vi "sensor_parser.vi"(0 "Sensor configuration":string, 2 "error in":errorcluster) -> (3 "include_annotation":bool, 4 "Port out":u16, 5 "Stream dimensions":cluster{"x dimension":i32, "y dimension":i32}, 6 "error out":errorcluster)   [LabVIEW 2025]
doc: "Gets Sensor type and ports from the configuration text."
panel:
  out "Sensor":string
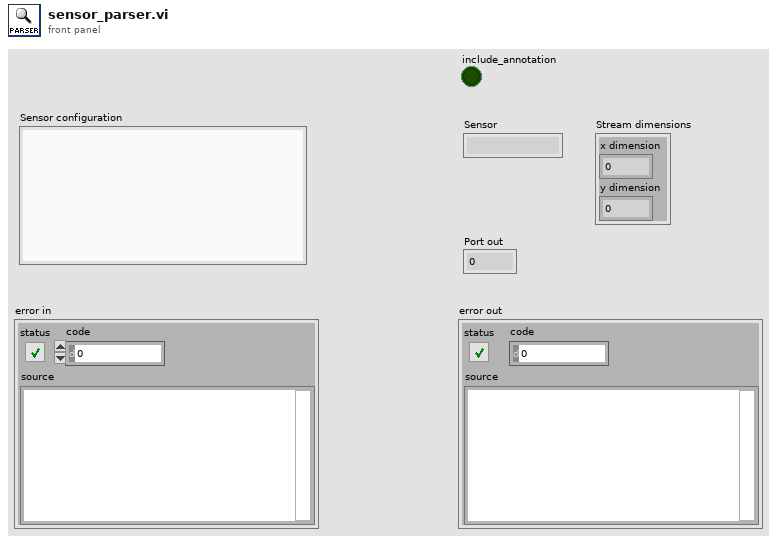
[diagram p1: front panel]
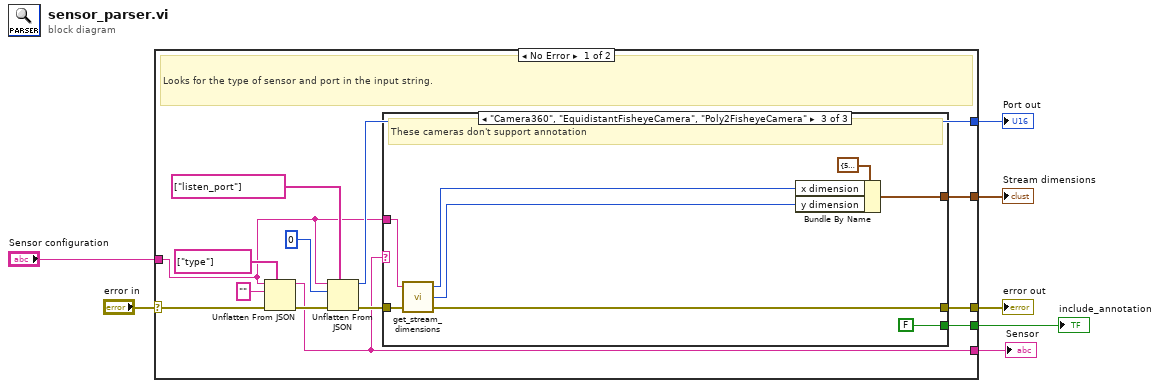
[diagram p0: block diagram]
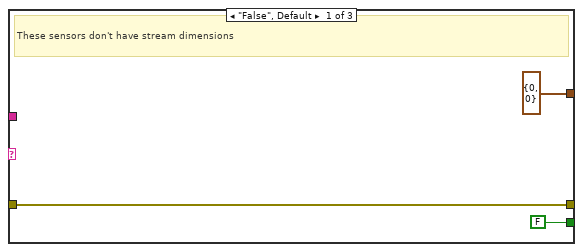
[diagram p2: hidden frame]
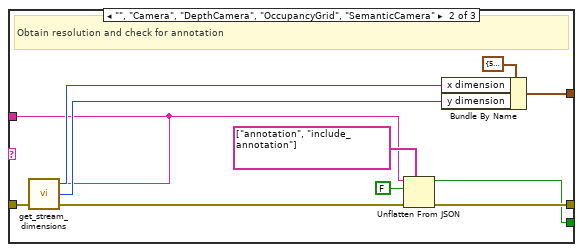
[diagram p3: hidden frame]
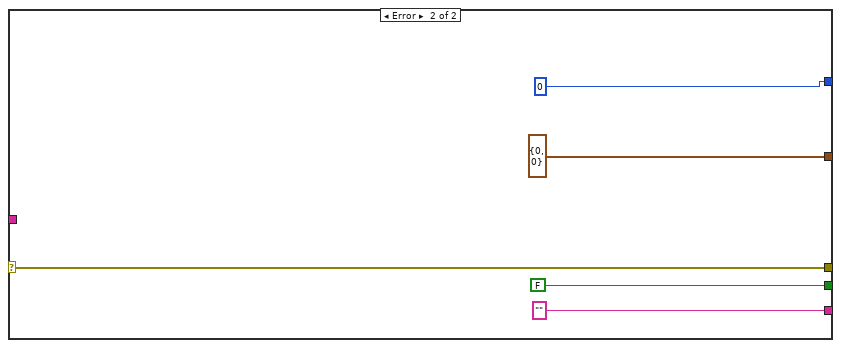
[diagram p4: hidden frame]
diagram:
  n1 = case shown="No Error" "error in" {
    selector: "error in" -> [w16 w47]
    tunnel: [w11 w47] -> w6
    tunnel: "Sensor configuration" -> [w9 _]
    tunnel: [w10 "" ("result string")] -> w4
    tunnel: [w13 u16 0] -> w3
    tunnel: [w20 cluster{"x dimension":i32, "y dimension":i32} {"x dimension"=0, "y dimension"=0} ("stream dimensions")] -> w2
    tunnel: [w8 FALSE] -> w1
    frame No Error {
      # "Looks for the type of sensor and port in the input string."
      n2 = Unflatten From JSON(path=string[] ["type"], JSON string=w9, type and defaults="", error in (no error)=w16) -> (value=w10:string, error out=w17:errorcluster)  [unwired: 3 in]
      n3 = Unflatten From JSON(path=string[] ["listen_port"], JSON string=w9, type and defaults=u16 0 ("Port"), error in (no error)=w17) -> (value=w13:u16, error out=w12:errorcluster)  [unwired: 3 in]
      n4 = case shown="\"Camera360\", \"EquidistantFisheyeCamera\", \"Poly2FisheyeCamera\"" w10 {
        tunnel: [cluster{"x dimension":i32, "y dimension":i32} {"x dimension"=0, "y dimension"=0} ("stream dimensions") w33 w41] -> w20
        tunnel: w9 -> [_ w27 w37]
        tunnel: w12 -> [w22 w32 w40]
        tunnel: [w22 w25 w36] -> w11
        tunnel: [FALSE w24 FALSE] -> w8
        frame "False", Default {
          # "These sensors don't have stream dimensions"
        }
        frame "", "Camera", "DepthCamera", "OccupancyGrid", "SemanticCamera" {
          # "Obtain resolution and check for annotation"
          n5 = call "get_stream_dimensions.vi"("error in"=w32, "Sensor configuration"=w27) -> ("error out"=w26:errorcluster, "y"=w30:i32, "x"=w31:i32)  [unwired: 1 in]
          n6 = Unflatten From JSON(path=string[] ["annotation", "include_annotation"], JSON string=w27, type and defaults=FALSE, error in (no error)=w26) -> (value=w24:bool, error out=w25:errorcluster)  [unwired: 3 in]
          n7 = Bundle By Name(cluster=cluster{"x dimension":i32, "y dimension":i32} {"x dimension"=512, "y dimension"=512} ("stream dimensions"), "x dimension"=w31, "y dimension"=w30) -> (w33:cluster{"x dimension":i32, "y dimension":i32})
        }
        frame "Camera360", "EquidistantFisheyeCamera", "Poly2FisheyeCamera" {
          # "These cameras don't support annotation"
          n8 = call "get_stream_dimensions.vi"("error in"=w40, "Sensor configuration"=w37) -> ("error out"=w36:errorcluster, "y"=w38:i32, "x"=w39:i32)  [unwired: 1 in]
          n9 = Bundle By Name(cluster=cluster{"x dimension":i32, "y dimension":i32} {"x dimension"=512, "y dimension"=512} ("stream dimensions"), "x dimension"=w39, "y dimension"=w38) -> (w41:cluster{"x dimension":i32, "y dimension":i32})
        }
      }
    }
    frame Error {
    }
  }
  "error out" <- w6
  "Sensor" <- w4
  "Port out" <- w3
  "Stream dimensions" <- w2
  "include_annotation" <- w1
